vi "showMessage.vi"(8 "error in (no error)":errorcluster, 11 "Instance In":refnum<data-value>) -> (0 "error out":errorcluster, 3 "Instance out":refnum<data-value>)   [LabVIEW 2017, in "SingleObject.lvclass"]
uses:
  SingleObject.lvclass
  SingleObject.lvclass/SingleObject.ctl
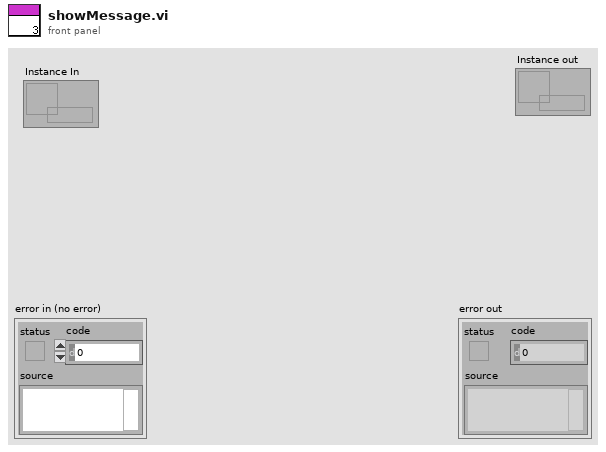
[diagram p1: front panel]
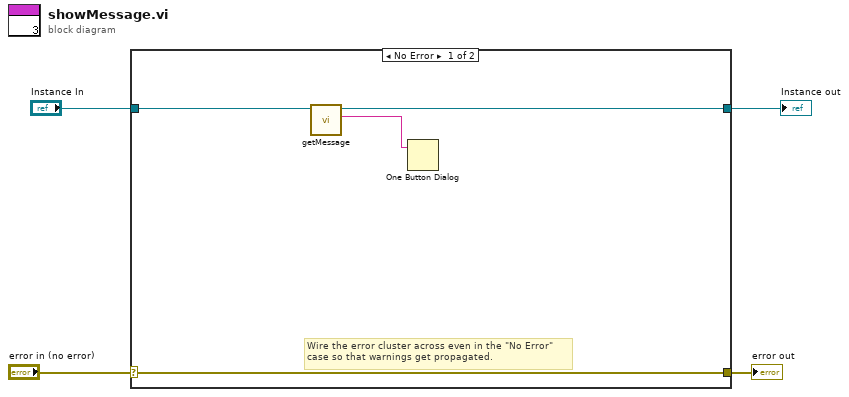
[diagram p0: block diagram]
diagram:
  n1 = case shown="No Error" "error in (no error)" {
    selector: "error in (no error)" -> [w8 w10]
    tunnel: [w8 w10] -> w3
    tunnel: "Instance In" -> [w7 w9]
    tunnel: [w6 w9] -> w1
    frame No Error {
      # "Wire the error cluster across even in the \"No Error\"\ncase so that warnings get propagated."
      n2 = call "getMessage.vi"("Instance In"=w7) -> ("Message"=w5:string, "Instance out"=w6:refnum<data-value>)  [unwired: 8 in, 1 out]
      n3 = One Button Dialog(message=w5) -> ()  [unwired: 1 in, 1 out]
    }
    frame Error {
    }
  }
  "error out" <- w3
  "Instance out" <- w1
